vi "ingest.tabular_set_timestamp_relative.vi"(8 "error in":errorcluster, 11 "TabularIngestStaging in":refnum<class "TabularIngestStaging.lvclass">) -> (0 "error out":errorcluster, 3 "TabularIngestStaging out":refnum<class "TabularIngestStaging.lvclass">)   [LabVIEW 2020, in "TabularIngestStaging.lvclass"]
doc: "Specifies that row timestamps are numeric offsets from a start time in the named column."
uses:
  TabularIngestStaging.lvclass
  TabularIngestStaging.lvclass/TabularIngestStaging.ctl
  client.lvlib
panel:
  in  "column":string
  in  "time_unit":i32
  in  "offset_ms":dbl
  in  "has_offset":bool
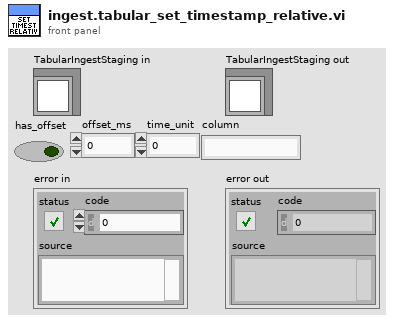
[diagram p1: front panel]
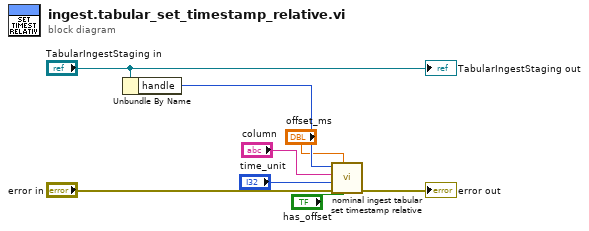
[diagram p0: block diagram]
diagram:
  n1 = Unbundle By Name("TabularIngestStaging in") -> ("handle"=w6:i32)
  n2 = call "nominal ingest tabular set timestamp relative.vi"("has_offset"="has_offset", "offset_ms"="offset_ms", "error in (no error)"="error in", "time_unit"="time_unit", "column"="column", "staging"=w6) -> ("error out"=→"error out":errorcluster)  [unwired: 4 in, 1 out]
  "TabularIngestStaging out" <- "TabularIngestStaging in"
